vi "Close Device Core.vi"(8 "error in (no error)":errorcluster, 11 "BNT_ULx-MCSV-DOPWM in":refnum<class "BNT_ULx-MCSV-DOPWM.lvclass">) -> (0 "error out":errorcluster, 3 "BNT_ULx-MCSV-DOPWM out":refnum<class "BNT_ULx-MCSV-DOPWM.lvclass">)   [LabVIEW 2021, in "BNT_ULx.lvlib" / "BNT_ULx-MCSV-DOPWM.lvclass"]
doc: "Close device driver connection."
uses:
  BNT_ULx-MCSV-DOPWM.lvclass
  C:/Users/Holger/Documents/LVP/CSPP/CSPP-Template/Packages/BNT_ULx/BNT_ULx-MCSV/BNT_ULx-MCSV.lvclass
  BNT_ULx-MCSV/BNT_ULx-MCSV.lvclass/BNT_ULx-MCSV.ctl
  BNT_ULx-MCSV/BNT_ULx-MCSV.lvclass
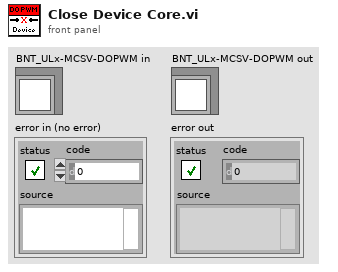
[diagram p1: front panel]
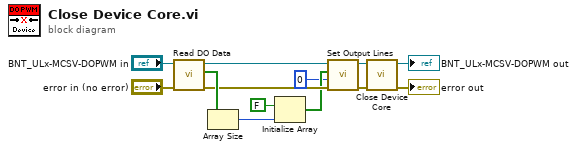
[diagram p0: block diagram]
diagram:
  n1 = call "Read DO Data.vi"("error in (no error)"="error in (no error)", "BNT_ULx-MCSV in"="BNT_ULx-MCSV-DOPWM in") -> ("error out"=w3:errorcluster, "DO Data"=w7:bool[], "BNT_ULx-MCSV out"=w6:refnum<class "BNT_ULx-MCSV-DOPWM.lvclass">)  [unwired: 7 in]
  n2 = Array Size(array=w7) -> (size(s)=w11:i32)
  n3 = Initialize Array(FALSE, w11) -> (w2:bool[])
  n4 = call "Set Output Lines.vi"("Error In"=w3, "Start Index"=0, "DO Lines"=w2, "BNT_ULx-MCSV in"=w6) -> ("Error Out"=w4:errorcluster, "BNT_ULx-MCSV out"=w5:refnum<class "BNT_ULx-MCSV-DOPWM.lvclass">)  [unwired: 6 in]
  n5 = call-parent "Close Device Core.vi"("error in (no error)"=w4, "BNT_ULx-MCSV in"=w5) -> ("error out"=→"error out":errorcluster, "BNT_ULx-MCSV out"=→"BNT_ULx-MCSV-DOPWM out":refnum<class "BNT_ULx-MCSV-DOPWM.lvclass">)  [unwired: 8 in]
